vi "Get Employee Info Names and Types Array.vi"(8 "error in (no error)":errorcluster caption="错误输入（无错误）", 11 "Employee 输入":refnum<class "Employee.lvclass"> caption="DNL_LabVIEW Object in") -> (0 "error out":errorcluster caption="错误输出", 1 "Colomn Types":variant[](array[variant]), 2 "Column Names":string[](array[string]), 3 "Employee 输出":refnum<class "Employee.lvclass"> caption="DNL_LabVIEW Object out")   [LabVIEW 2012, in "Employee.lvclass"]
uses:
  Employee.lvclass
  Custom Def/Employee Info.ctl
panel:
  in  "Employee Info":T1
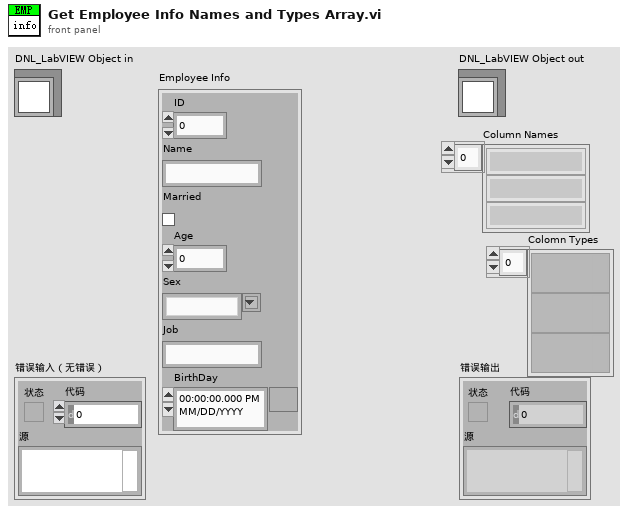
[diagram p1: front panel]
types:
  T1 = typedef "Employee Info.ctl" = cluster{"ID":u16, "Name":string, "Married":bool, "Age":u8, "Sex":string, "Job":string, "BirthDay":timestamp}
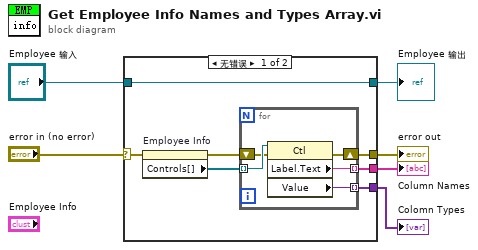
[diagram p0: block diagram]
diagram:
  n1 = case shown="无错误" "error in (no error)" {
    selector: "error in (no error)" -> [w9 w20]
    tunnel: [w12 w20] -> w5
    tunnel: [w13 w19] -> w3
    tunnel: "Employee 输入" -> [w13 w19]
    tunnel: [w11 _] -> w2
    tunnel: [w10 _] -> w1
    frame No Error {
      n2 = property on="Employee Info" class="Clust (严格)"(error in=w9) -> (error out=w8:errorcluster, "Controls[]"=w7:refnum<vi>[])  [unwired: 1 in, 1 out]
      n3 = for {
        tunnel: w7 -> [w18] mode=indexing
        tunnel: [w17] -> w11 mode=indexing
        tunnel: [w16] -> w10 mode=indexing
        shift-right: [w14] -> w12
        shift-left: w8 -> [w15]
        n4 = property class="Ctl"(reference=w18, error in=w15) -> (error out=w14:errorcluster, "Label.Text"=w17:string, "Value"=w16:variant)  [unwired: 1 out]
      }
    }
    frame Error {
    }
  }
  "error out" <- w5
  "Employee 输出" <- w3
  "Colomn Types" <- w1
  "Column Names" <- w2
